vi "Using a Queue As a Multiplexer.vi"() -> ()   [LabVIEW 2023]
doc: "This VI shows the similarity between Queues and multiplexers. Multiplex means \"many-to-one\". Queues allow data to be sent to one location from many data sources. In this VI, three loops generate sine data, and one loop consumes the data, and all of them run in parallel."
panel:
  out "Waveform Chart":dbl(graph)
  in  "Stop":bool
  # "Overview: Demonstrates the use of the Queue functions to implement a multiplexer.\nInstructions:\nRun the VI."
  # "The data for this single chart is being generated by three parallel loops."
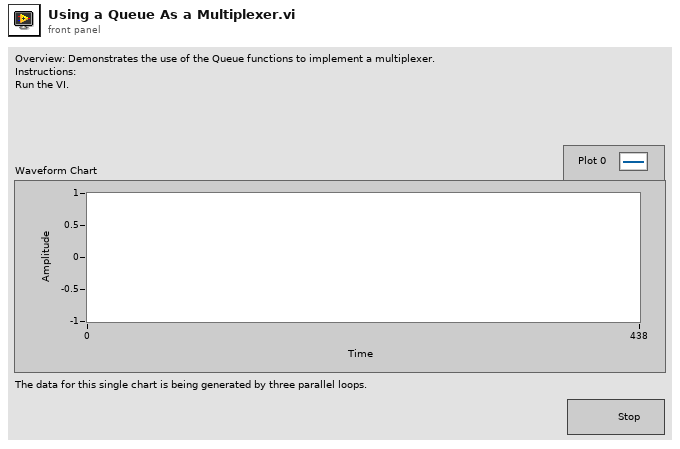
[diagram p1: front panel]
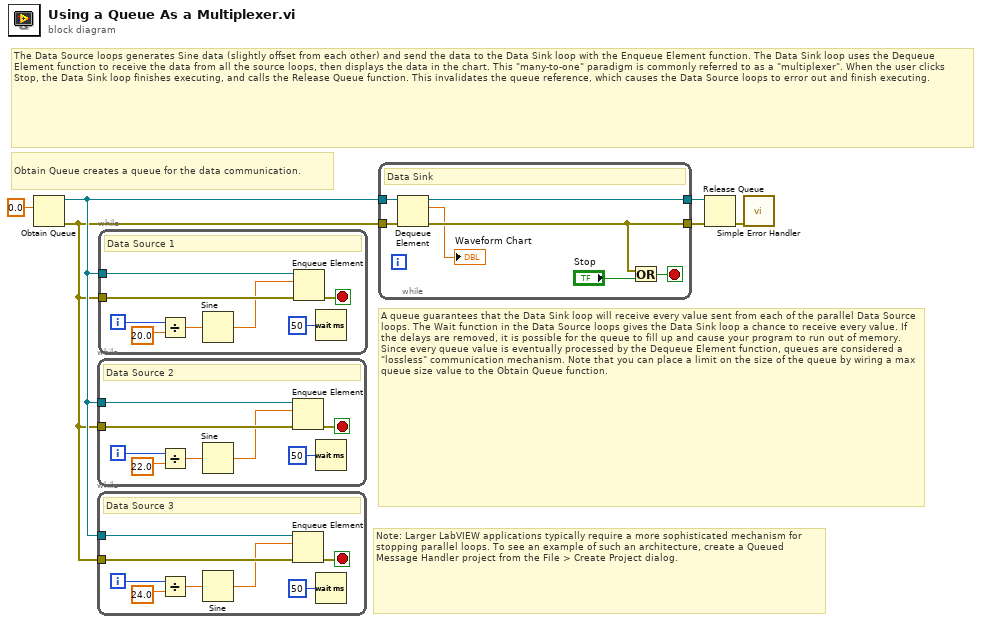
[diagram p0: block diagram]
diagram:
  # "Note: Larger LabVIEW applications typically require a more sophisticated mechanism for stopping parallel loops. To see an example of such an architecture, create a Queued Message Handler project from the File > Create Project dialog."
  # "Obtain Queue creates a queue for the data communication."
  # "The Data Source loops generates Sine data (slightly offset from each other) and send the data to the Data Sink loop with the Enqueue Element function. The Data Sink loop uses the Dequeue Element function to receive the data from all the source loops, then displays the data in the chart. This \"many-to-one\" paradigm is commonly referred to as a \"multiplexer\". When the user clicks Stop, the Data Sink loop finishes executing, and calls the Release Queue function. This invalidates the queue reference, which causes the Data Source loops to error out and finish executing."
  # "A queue guarantees that the Data Sink loop will receive every value sent from each of the parallel Data Source loops. The Wait function in the Data Source loops gives the Data Sink loop a chance to receive every value. If the delays are removed, it is possible for the queue to fill up and cause your program to run out of memory. Since every queue value is eventually processed by the Dequeue Element function, queues are considered a \"lossless\" communication mechanism. Note that you can place a limit on the size of the queue by wiring a max queue size value to the Obtain Queue function."
  n1 = Obtain Queue(element data type=0.0) -> (queue out=w2:refnum<queue>, error out=w1:errorcluster)  [unwired: 4 in, 1 out]
  n2 = while "Data Sink One" {
    tunnel: w2 -> [w14]
    tunnel: w1 -> [w13]
    i -> [w10]
    stop <- w12 stop-if-true
    # "Data Source 2"
    n3 = Divide(x=w10, y=22.0) -> (x/y=w11:dbl)
    n4 = Sine(x=w11) -> (sin(x)=w8:dbl)
    n5 = Enqueue Element(queue=w14, element=w8, error in (no error)=w13) -> (error out=w12:errorcluster)  [unwired: 1 in, 2 out]
    n6 = Wait (ms)(milliseconds to wait=u32 50) -> ()  [unwired: 1 out]
  }
  n7 = while "Data Sink One" {
    tunnel: w2 -> [w22]
    tunnel: w1 -> [w21]
    i -> [w18]
    stop <- w20 stop-if-true
    # "Data Source 3"
    n8 = Divide(x=w18, y=24.0) -> (x/y=w19:dbl)
    n9 = Sine(x=w19) -> (sin(x)=w16:dbl)
    n10 = Enqueue Element(queue=w22, element=w16, error in (no error)=w21) -> (error out=w20:errorcluster)  [unwired: 1 in, 2 out]
    n11 = Wait (ms)(milliseconds to wait=u32 50) -> ()  [unwired: 1 out]
  }
  n12 = while "Data Sink One" {
    tunnel: w2 -> [w30]
    tunnel: w1 -> [w29]
    i -> [w27]
    stop <- w28 stop-if-true
    # "Data Source 1"
    n13 = Divide(x=w27, y=20.0) -> (x/y=w26:dbl)
    n14 = Sine(x=w26) -> (sin(x)=w24:dbl)
    n15 = Enqueue Element(queue=w30, element=w24, error in (no error)=w29) -> (error out=w28:errorcluster)  [unwired: 1 in, 2 out]
    n16 = Wait (ms)(milliseconds to wait=u32 50) -> ()  [unwired: 1 out]
  }
  n17 = while "Data Source Loop" {
    tunnel: w2 -> [w37]
    tunnel: w1 -> [w36]
    tunnel: [w34] -> w6
    tunnel: [w32] -> w5
    stop <- w33 stop-if-true
    # "Data Sink"
    n18 = Dequeue Element(queue=w37, error in (no error)=w36) -> (queue out=w34:refnum<queue>, element=→"Waveform Chart":dbl, error out=w32:errorcluster)  [unwired: 1 in, 1 out]
    n19 = Or(x=w32, y="Stop") -> (x .or. y?=w33:bool)
  }
  n20 = Release Queue(queue=w6, error in (no error)=w5) -> (error out=w3:errorcluster)  [unwired: 1 in, 2 out]
  n21 = call <vilib>:"Simple Error Handler.vi"("error in (no error)"=w3) -> ()  [unwired: 4 in, 5 out]
